vi "Update Value Control_.vi"(8 "error in (no error)":errorcluster, 9 "Tab Control Ref In":T2, 10 "Attirbutes":T1[](array[typedef]), 11 "Tree Control In":refnum<vi>) -> (0 "error out":errorcluster, 1 "Tooltip":string, 2 "Units":string)   [LabVIEW 2020, in "Camera Settings Dialog UI.lvlib" / "Camera Settings Dialog.lvclass"]
doc: "The Update Value Control subVI determines the type of the attribute selected, displays the corresponding tab in the tab control, sets the current value of the control, sets the minimum and maximum of the control (for numerics), and disables the control if the attribute is not writables."
uses:
  Camera Settings Dialog.lvclass
  Camera Attribute Info.ctl
  Attribute Type.ctl
  Camera Settings Dialog.lvclass/Camera Settings Dialog.ctl
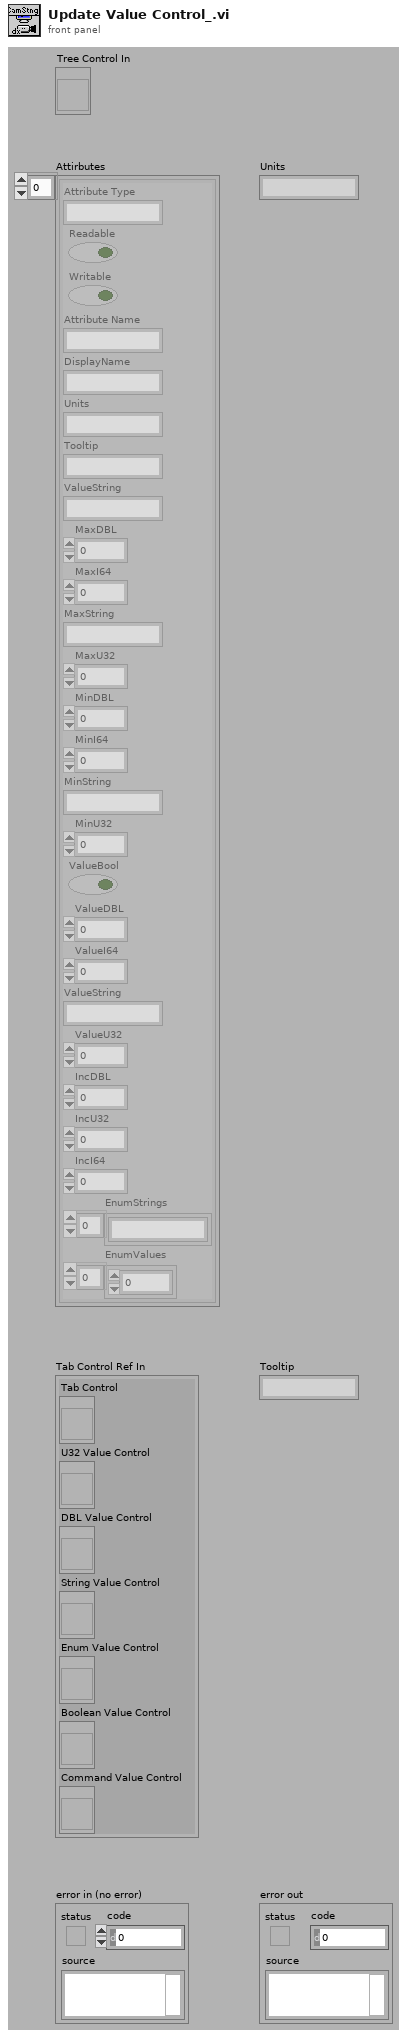
[diagram p1: front panel]
types:
  T1 = typedef "Camera Attribute Info.ctl" = cluster{"Attribute Type":string, "Readable":bool, "Writable":bool, "Attribute Name":string, "DisplayName":string, "Units":string, "Tooltip":string, "ValueString":string, "MaxDBL":dbl, "MaxI64":i64, "MaxString":string, "MaxU32":u32, "MinDBL":dbl, "MinI64":i64, "MinString":string, "MinU32":u32, "ValueBool":bool, "ValueDBL":dbl, "ValueI64 ":i64, "ValueString":string, "ValueU32":u32, "IncDBL":dbl, "IncU32":u32, "IncI64":i64, "EnumStrings":string[], "EnumValues":u32[]}
  T2 = cluster{"Tab Control":refnum<vi>, "U32 Value Control":refnum<vi>, "DBL Value Control":refnum<vi>, "String Value Control":refnum<vi>, "Enum Value Control":refnum<vi>, "Boolean Value Control":refnum<vi>, "Command Value Control":refnum<vi>}
  T3 = enum32{"U32", "DBL", "String", "Enum", "Bool", "Command"}
  T4 = typedef "Attribute Type.ctl" = enum32{"U32", "I64", "DBL", "String", "Enum", "Bool", "Command"}
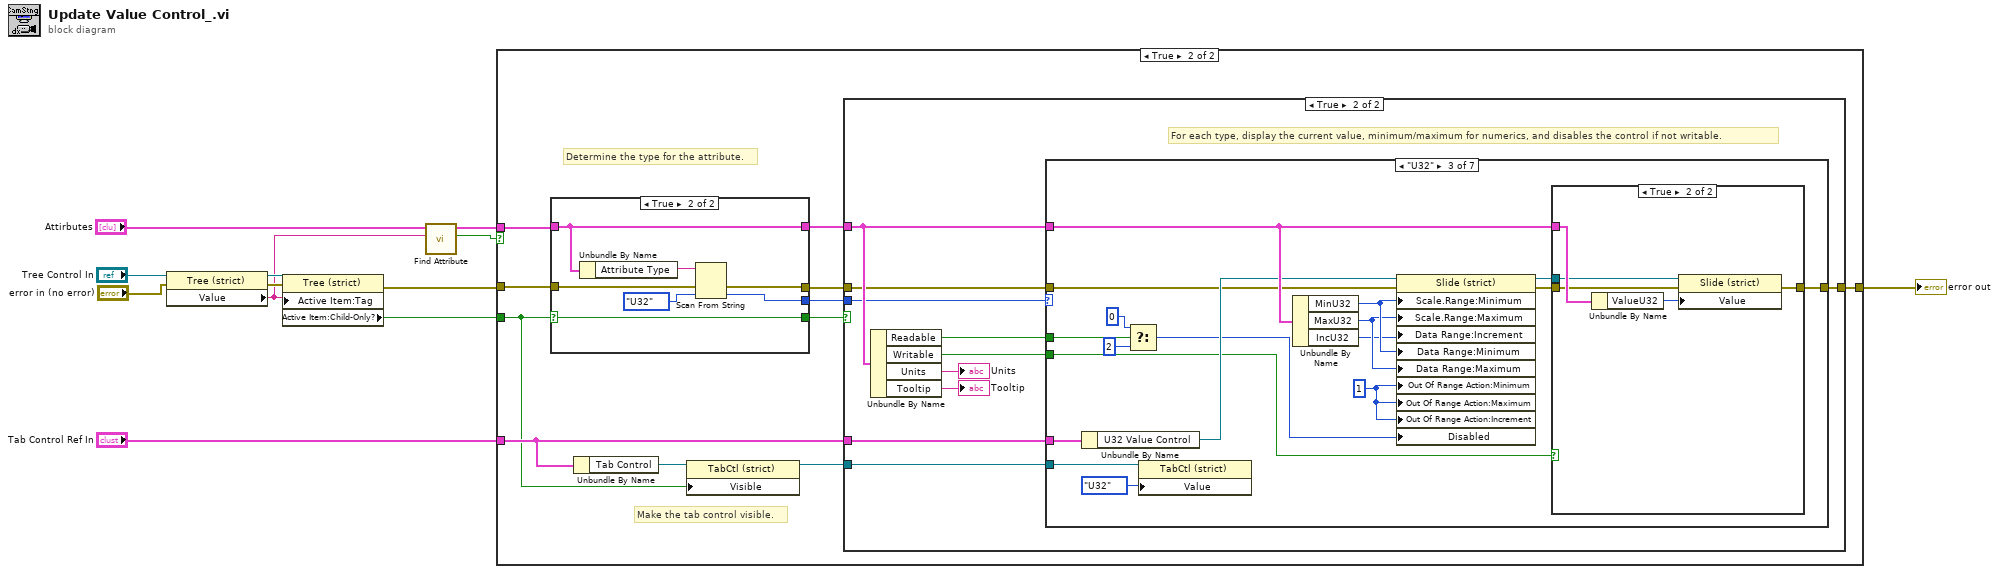
[diagram p0: block diagram]
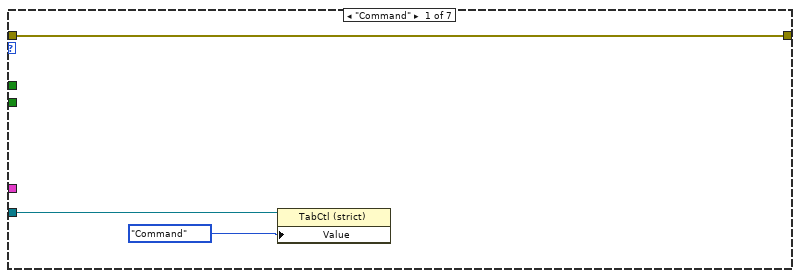
[diagram p4: hidden frame]
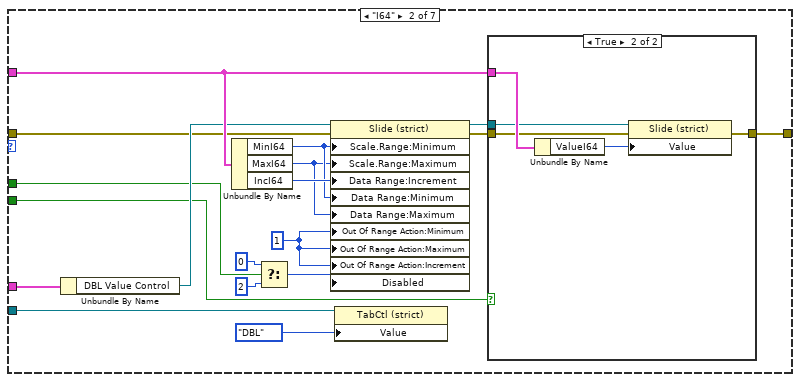
[diagram p5: hidden frame]
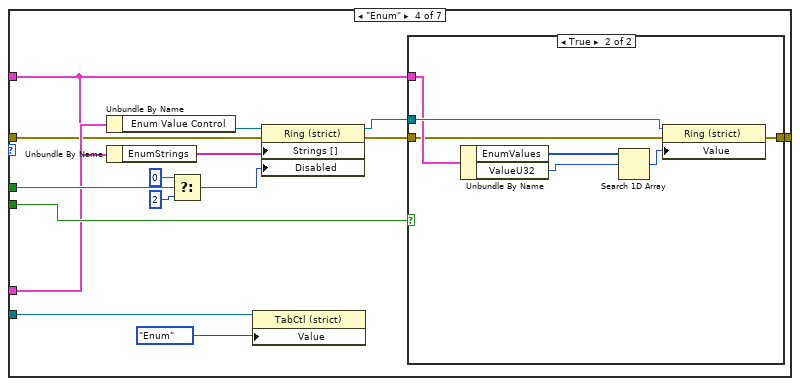
[diagram p8: hidden frame]
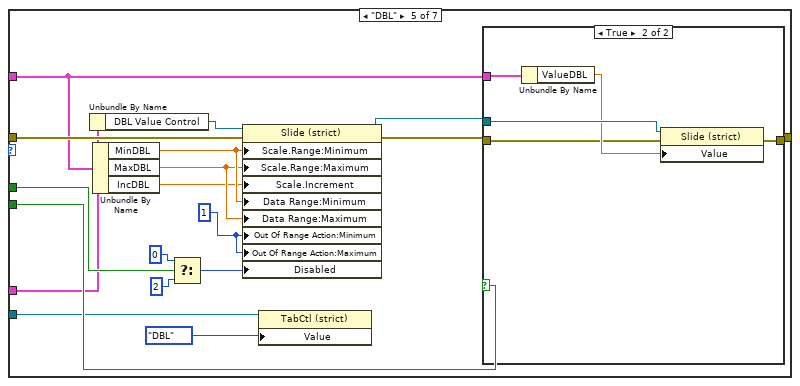
[diagram p10: hidden frame]
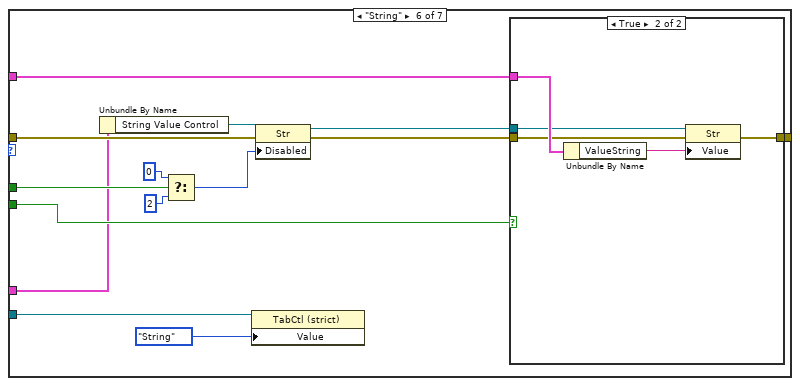
[diagram p12: hidden frame]
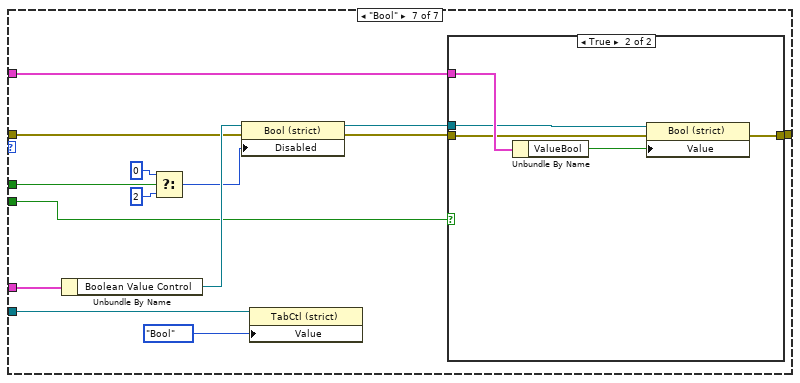
[diagram p14: hidden frame]
diagram:
  n1 = property class="Tree (strict)"(reference="Tree Control In", error in="error in (no error)") -> (reference out=w11:refnum<vi>, error out=w10:errorcluster, "Value"=w5:string)
  n2 = property class="Tree (strict)"(reference=w11, error in=w10, "Active Item:Tag"=w5) -> (error out=w1:errorcluster, "Active Item:Child-Only?"=w7:bool)  [unwired: 1 out]
  n3 = call "Find Attribute.vi"("Attr Name"=w5, "Attirbutes"="Attirbutes") -> ("Found?"=w4:bool, "Attribute Information"=w3:T1)  [unwired: 8 in]
  n4 = case shown="True" w4 {
    tunnel: w1 -> [w13 w21]
    tunnel: [w13 w20] -> w12
    tunnel: "Tab Control Ref In" -> [_ w24]
    tunnel: w7 -> [_ w14]
    tunnel: w3 -> [_ w17]
    frame False {
    }
    frame True {
      # "Make the tab control visible."
      # "Determine the type for the attribute."
      n5 = case shown="True" w14 {
        selector: w14 -> [w174 w177]
        tunnel: [_ w181] -> w22
        tunnel: w21 -> [w176 w179]
        tunnel: [w176 w180] -> w23
        tunnel: w17 -> [w175 w178]
        tunnel: [w175 w178] -> w16
        tunnel: [w174 w177] -> w15
        frame False {
        }
        frame True {
          n6 = Unbundle By Name(w178) -> ("Attribute Type"=w182:string)
          n7 = Scan From String(input string=w182, error in=w179, default 1=Attribute_Type."U32" ("Attribute Type")) -> (error out=w180:errorcluster, output 1=w181:T4)  [unwired: 2 in, 2 out]
        }
      }
      n8 = Unbundle By Name(w24) -> ("Tab Control"=w19:refnum<vi>)
      n9 = property class="TabCtl (strict)"(reference=w19, "Visible"=w14) -> (reference out=w18:refnum<vi>)  [unwired: 1 in, 1 out]
      n10 = case shown="True" w15 {
        tunnel: w23 -> [w25 w33]
        tunnel: [w25 w31] -> w20
        tunnel: w22 -> [_ w32]
        tunnel: w24 -> [_ w35]
        tunnel: w18 -> [_ w30]
        tunnel: w16 -> [_ w34]
        frame False {
        }
        frame True {
          # "For each type, display the current value, minimum/maximum for numerics, and disables the control if not writable."
          n11 = Unbundle By Name(w34) -> ("Readable"=w29:bool, "Writable"=w28:bool, "Units"=→"Units":string, "Tooltip"=→"Tooltip":string)
          n12 = case shown="\"U32\"" w32 {
            tunnel: w29 -> [_ w53 w78 w101 w126 w146 w165]
            tunnel: w28 -> [_ w52 w77 w100 w125 w145 w164]
            tunnel: w34 -> [_ w56 w80 w87 w110 w144 w163]
            tunnel: w33 -> [w38 w39 w66 w88 w127 w147 w166]
            tunnel: [w38 w50 w75 w98 w123 w142 w161] -> w31
            tunnel: w35 -> [_ w54 w72 w95 w122 w140 w159]
            tunnel: w30 -> [w37 w49 w73 w96 w120 w141 w160]
            frame "Command" {
              n13 = property class="TabCtl (strict)"(reference=w37, "Value"=T3."Command" ("Tab Control")) -> ()  [unwired: 1 in, 2 out]
            }
            frame "I64" {
              w40 = u8 1 ("Response to Value Outside Limits:Minimum")
              n14 = Unbundle By Name(w54) -> ("DBL Value Control"=w55:refnum<vi>)
              n15 = Unbundle By Name(w56) -> ("MinI64"=w42:i64, "MaxI64"=w41:i64, "IncI64"=w43:i64)
              n16 = Select(t=0, s=w53, f=2) -> (s? t:f=w44:i32)
              n17 = property class="Slide (strict)"(reference=w55, error in=w39, "Scale.Range:Minimum"=w42, "Scale.Range:Maximum"=w41, "Data Range:Increment"=w43, "Data Range:Minimum"=w42, "Data Range:Maximum"=w41, "Out Of Range Action:Minimum"=w40, "Out Of Range Action:Maximum"=w40, "Out Of Range Action:Increment"=w40, "Disabled"=w44) -> (reference out=w48:refnum<vi>, error out=w51:errorcluster)
              n18 = property class="TabCtl (strict)"(reference=w49, "Value"=T3."DBL" ("Tab Control")) -> ()  [unwired: 1 in, 2 out]
              n19 = case shown="True" w52 {
                tunnel: w56 -> [_ w62]
                tunnel: w51 -> [w57 w58]
                tunnel: [w57 w61] -> w50
                tunnel: w48 -> [_ w60]
                frame False {
                }
                frame True {
                  n20 = Unbundle By Name(w62) -> ("ValueI64"=w59:i64)
                  n21 = property class="Slide (strict)"(reference=w60, error in=w58, "Value"=w59) -> (error out=w61:errorcluster)  [unwired: 1 out]
                }
              }
            }
            frame "U32" {
              w67 = u8 1 ("Out Of Range Action:Maximum")
              n22 = Unbundle By Name(w72) -> ("U32 Value Control"=w79:refnum<vi>)
              n23 = Select(t=0, s=w78, f=2) -> (s? t:f=w69:i32)
              n24 = property class="TabCtl (strict)"(reference=w73, "Value"=T3."U32" ("Tab Control")) -> ()  [unwired: 1 in, 2 out]
              n25 = Unbundle By Name(w80) -> ("MinU32"=w65:u32, "MaxU32"=w64:u32, "IncU32"=w63:u32)
              n26 = property class="Slide (strict)"(reference=w79, error in=w66, "Scale.Range:Minimum"=w65, "Scale.Range:Maximum"=w64, "Data Range:Increment"=w63, "Data Range:Minimum"=w65, "Data Range:Maximum"=w64, "Out Of Range Action:Minimum"=w67, "Out Of Range Action:Maximum"=w67, "Out Of Range Action:Increment"=w67, "Disabled"=w69) -> (reference out=w74:refnum<vi>, error out=w76:errorcluster)
              n27 = case shown="True" w77 {
                tunnel: w76 -> [w81 w85]
                tunnel: [w81 w83] -> w75
                tunnel: w74 -> [_ w84]
                tunnel: w80 -> [_ w86]
                frame False {
                }
                frame True {
                  n28 = Unbundle By Name(w86) -> ("ValueU32"=w82:u32)
                  n29 = property class="Slide (strict)"(reference=w84, error in=w85, "Value"=w82) -> (error out=w83:errorcluster)  [unwired: 1 out]
                }
              }
            }
            frame "Enum" {
              n30 = Unbundle By Name(w95) -> ("Enum Value Control"=w94:refnum<vi>)
              n31 = Unbundle By Name(w87) -> ("EnumStrings"=w89:string[])
              n32 = Select(t=0, s=w101, f=2) -> (s? t:f=w91:i32)
              n33 = property class="TabCtl (strict)"(reference=w96, "Value"=T3."Enum" ("Tab Control")) -> ()  [unwired: 1 in, 2 out]
              n34 = property class="Ring (strict)"(reference=w94, error in=w88, "Strings []"=w89, "Disabled"=w91) -> (reference out=w97:refnum<vi>, error out=w99:errorcluster)
              n35 = case shown="True" w100 {
                tunnel: w99 -> [w102 w104]
                tunnel: [w102 w109] -> w98
                tunnel: w97 -> [_ w107]
                tunnel: w87 -> [_ w106]
                frame False {
                }
                frame True {
                  n36 = Unbundle By Name(w106) -> ("EnumValues"=w105:u32[], "ValueU32"=w103:u32)
                  n37 = Search 1D Array(1D array=w105, element=w103) -> (index of element=w108:i32)  [unwired: 1 out]
                  n38 = property class="Ring (strict)"(reference=w107, error in=w104, "Value"=w108) -> (error out=w109:errorcluster)  [unwired: 1 out]
                }
              }
            }
            frame "DBL" {
              w114 = u8 1 ("Out Of Range Action:Minimum")
              n39 = Unbundle By Name(w122) -> ("DBL Value Control"=w121:refnum<vi>)
              n40 = Unbundle By Name(w110) -> ("MinDBL"=w113:dbl, "MaxDBL"=w112:dbl, "IncDBL"=w111:dbl)
              n41 = Select(t=0, s=w126, f=2) -> (s? t:f=w116:i32)
              n42 = property class="Slide (strict)"(reference=w121, error in=w127, "Scale.Range:Minimum"=w113, "Scale.Range:Maximum"=w112, "Scale.Increment"=w111, "Data Range:Minimum"=w113, "Data Range:Maximum"=w112, "Out Of Range Action:Minimum"=w114, "Out Of Range Action:Maximum"=w114, "Disabled"=w116) -> (reference out=w119:refnum<vi>, error out=w124:errorcluster)
              n43 = property class="TabCtl (strict)"(reference=w120, "Value"=T3."DBL" ("Tab Control")) -> ()  [unwired: 1 in, 2 out]
              n44 = case shown="True" w125 {
                tunnel: w124 -> [w128 w129]
                tunnel: [w128 w133] -> w123
                tunnel: w119 -> [_ w132]
                tunnel: w110 -> [_ w131]
                frame False {
                }
                frame True {
                  n45 = Unbundle By Name(w131) -> ("ValueDBL"=w130:dbl)
                  n46 = property class="Slide (strict)"(reference=w132, error in=w129, "Value"=w130) -> (error out=w133:errorcluster)  [unwired: 1 out]
                }
              }
            }
            frame "String" {
              n47 = Unbundle By Name(w140) -> ("String Value Control"=w139:refnum<vi>)
              n48 = Select(t=0, s=w146, f=2) -> (s? t:f=w134:i32)
              n49 = property class="TabCtl (strict)"(reference=w141, "Value"=T3."String" ("Tab Control")) -> ()  [unwired: 1 in, 2 out]
              n50 = property class="Str"(reference=w139, error in=w147, "Disabled"=w134) -> (reference out=w138:refnum<vi>, error out=w143:errorcluster)
              n51 = case shown="True" w145 {
                tunnel: w144 -> [_ w153]
                tunnel: w143 -> [w148 w149]
                tunnel: [w148 w152] -> w142
                tunnel: w138 -> [_ w151]
                frame False {
                }
                frame True {
                  n52 = Unbundle By Name(w153) -> ("ValueString"=w150:string)
                  n53 = property class="Str"(reference=w151, error in=w149, "Value"=w150) -> (error out=w152:errorcluster)  [unwired: 1 out]
                }
              }
            }
            frame "Bool" {
              n54 = Unbundle By Name(w159) -> ("Boolean Value Control"=w167:refnum<vi>)
              n55 = Select(t=0, s=w165, f=2) -> (s? t:f=w154:i32)
              n56 = property class="Bool (strict)"(reference=w167, error in=w166, "Disabled"=w154) -> (reference out=w158:refnum<vi>, error out=w162:errorcluster)
              n57 = property class="TabCtl (strict)"(reference=w160, "Value"=T3."Bool" ("Tab Control")) -> ()  [unwired: 1 in, 2 out]
              n58 = case shown="True" w164 {
                tunnel: w163 -> [_ w173]
                tunnel: w162 -> [w168 w170]
                tunnel: [w168 w172] -> w161
                tunnel: w158 -> [_ w171]
                frame False {
                }
                frame True {
                  n59 = Unbundle By Name(w173) -> ("ValueBool"=w169:bool)
                  n60 = property class="Bool (strict)"(reference=w171, error in=w170, "Value"=w169) -> (error out=w172:errorcluster)  [unwired: 1 out]
                }
              }
            }
          }
        }
      }
    }
  }
  "error out" <- w12
